vi "main.vi"() -> ()   [LabVIEW 2015]
uses:
  <vilib>/measure/NI_MAPro.lvlib
  <vilib>/Analysis/NI_AALBase.lvlib
  <vilib>/measure/mamon.llb/Waveform Peak Detection for 1 Chan.vi
  <vilib>/Analysis/baseanly.llb/Mean (DBL).vi
  <vilib>/Instr/_visa.llb/VISA Configure Serial Port (Instr).vi
panel:
  out "Heart Rate":string
  in  "Force Redraw":bool
  out "read buffer":string
  out "error out":errorcluster
  out "Value of last sample":i32
  out "Heart Rate Plot":i32(graph)
  out "Main loop interations":i32
  in  "stop":bool
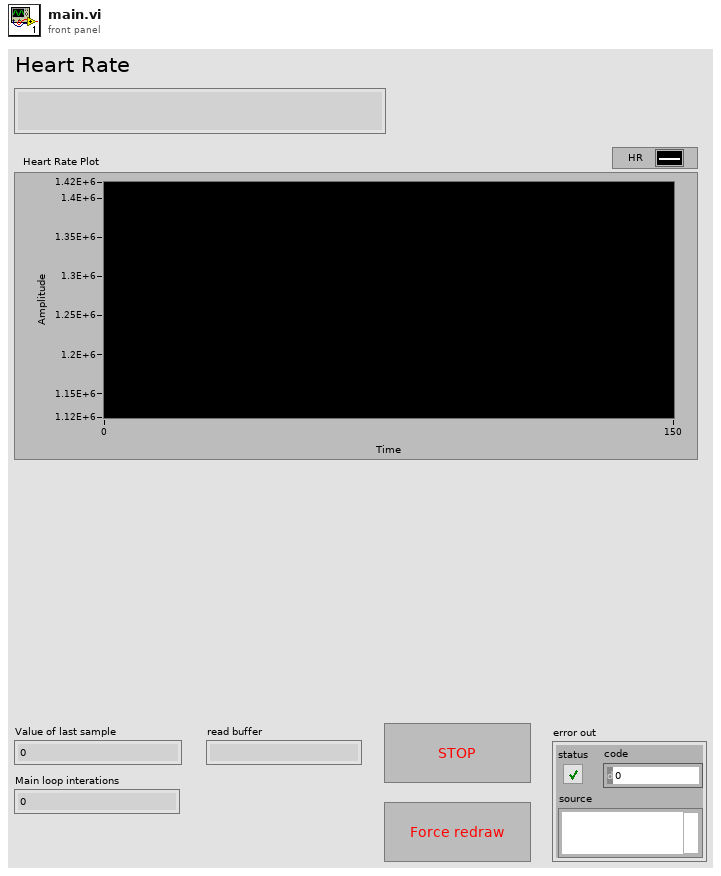
[diagram p1: front panel]
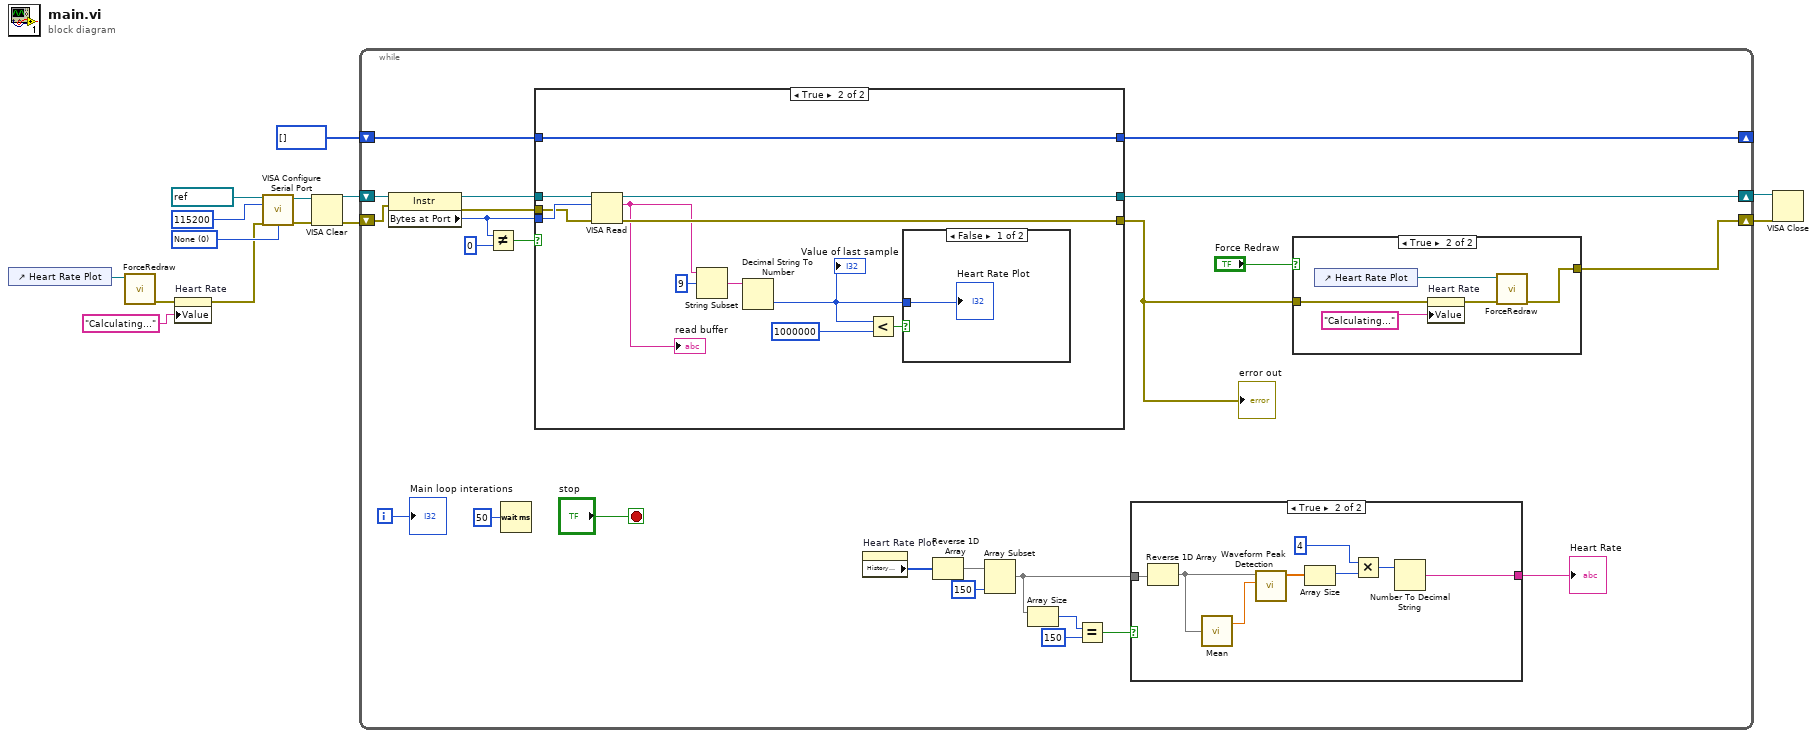
[diagram p0: block diagram]
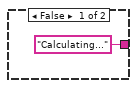
[diagram p2: hidden frame]
diagram:
  w10 = u16 0 items=["None", "XON/XOFF", "RTS/CTS", "XON/XOFF & RTS/CTS", "DTR/DSR", "XON/XOFF & DTR/DSR"] ("flow control (0:none)")
  n1 = control-ref of="Heart Rate Plot"() -> (w4:refnum<vi>)
  n2 = call "ForceRedraw.vi"("Waveform Chart ref"=w4) -> ("error out"=w3:errorcluster)  [unwired: 10 in]
  n3 = property on="Heart Rate" class="Str"(error in=w3, "Value"="Calculating..." ("Heart Rate")) -> (error out=w2:errorcluster)  [unwired: 1 in, 1 out]
  n4 = call-poly "VISA Configure Serial Port"("VISA resource name"=refnum<visa-resource-name> "COM3", "baud rate (9600)"=u32 115200, "error in (no error)"=w2, "flow control (0:none)"=w10) -> ("VISA resource name out"=w7:refnum<visa-resource-name>, "error out"=w6:errorcluster)  [unwired: 10 in]
  n5 = VISA Clear(VISA resource name=w7, error in (no error)=w6) -> (VISA resource name out=w8:refnum<visa-resource-name>, error out=w9:errorcluster)
  n6 = while {
    shift-right: [w37] -> w12
    shift-left: w8 -> [w36]
    shift-right: [w24] -> w11
    shift-left: w9 -> [w34]
    shift-right: [w26] -> _
    shift-left: i32[] [] -> [w29]
    i -> [w33]
    stop <- "stop" stop-if-true
    n7 = property class="Instr"(reference=w36, error in=w34) -> (reference out=w32:refnum<visa-resource-name>, error out=w35:errorcluster, "Bytes at Port"=w28:u32)
    n8 = Not Equal?(x=w28, y=u32 0) -> (x != y?=w30:bool)
    n9 = Wait (ms)(milliseconds to wait=u32 50) -> ()  [unwired: 1 out]
    n10 = case shown="True" w30 {
      tunnel: [w56 w68] -> w37
      tunnel: w28 -> [_ w67]
      tunnel: w35 -> [w55 w66]
      tunnel: [w55 w65] -> w23
      tunnel: w32 -> [w56 w64]
      tunnel: w29 -> [w54 w57]
      tunnel: [w54 w57] -> w26
      frame False {
      }
      frame True {
        n11 = VISA Read(VISA resource name=w64, byte count=w67, error in (no error)=w66) -> (VISA resource name out=w68:refnum<visa-resource-name>, read buffer=w62:string, error out=w65:errorcluster)  [unwired: 1 out]
        "read buffer" <- w62
        n12 = String Subset(string=w62, offset (0)=9) -> (substring=w61:string)  [unwired: 1 in]
        n13 = Decimal String To Number(string=w61) -> (number=w60:i32)  [unwired: 2 in, 1 out]
        "Value of last sample" <- w60
        n14 = Less?(x=w60, y=1000000) -> (x < y?=w58:bool)
        n15 = case shown="False" w58 {
          tunnel: w60 -> [w69 _]
          frame False {
            "Heart Rate Plot" <- w69
          }
          frame True {
          }
        }
      }
    }
    "error out" <- w23
    n16 = property on="Heart Rate Plot" class="WFChart (strict)"() -> ("History Data"=w22:i32[])  [unwired: 2 in, 2 out]
    n17 = Reverse 1D Array(array=w22) -> (reversed array=w21:i32[])
    n18 = Array Subset(array=w21, length=150) -> (w18:i32[])  [unwired: 1 in]
    n19 = Array Size(array=w18) -> (size(s)=w17:i32)
    n20 = Equal?(x=w17, y=150) -> (x = y?=w19:bool)
    n21 = case shown="True" w19 {
      tunnel: w18 -> [_ w44]
      tunnel: ["Calculating..." w40] -> w15
      frame False {
      }
      frame True {
        n22 = Reverse 1D Array(array=w44) -> (reversed array=w43:i32[])
        n23 = call-poly <vilib>:"Mean.vi"("X"=w43) -> ("mean"=w42:dbl)  [unwired: 1 out]
        n24 = call-poly <vilib>:"Waveform Peak Detection.vi"("threshold"=w42, "Signal In"=w43) -> ("Locations"=w47:dbl[])  [unwired: 5 in, 4 out]
        n25 = Array Size(array=w47) -> (size(s)=w46:i32)
        n26 = Multiply(x=4, y=w46) -> (x*y=w41:i32)
        n27 = Number To Decimal String(number=w41) -> (decimal integer string=w40:string)  [unwired: 1 in]
      }
    }
    "Heart Rate" <- w15
    n28 = case shown="True" "Force Redraw" {
      tunnel: [w48 w52] -> w24
      tunnel: w23 -> [w48 w50]
      frame False {
      }
      frame True {
        n29 = control-ref of="Heart Rate Plot"() -> (w53:refnum<vi>)
        n30 = property on="Heart Rate" class="Str"(error in=w50, "Value"="Calculating..." ("Heart Rate")) -> (error out=w49:errorcluster)  [unwired: 1 in, 1 out]
        n31 = call "ForceRedraw.vi"("error in"=w49, "Waveform Chart ref"=w53) -> ("error out"=w52:errorcluster)  [unwired: 9 in]
      }
    }
    "Main loop interations" <- w33
  }
  n32 = VISA Close(VISA resource name=w12, error in (no error)=w11) -> ()  [unwired: 1 out]
